vi "Open Playback Files Cropping.vi"(8 "error in (no error)":errorcluster, 11 "Frame Grabber Data In":T1={"Camera Session"="", "Frame"=refnum, "AVI Refnum"=refnum, "Codecs"=[], "Frame number"=0, "Tracking File Refnum"=refnum, "Tick Count"=0, "Probe Object"=refnum, "Playback Probe Data"=[], "Rigid Body"={"Position"={"x (mm)"=0.0, "y (mm)"=0.0, "z (mm)"=0.0}, "Orientation"={"Pitch (rad)"=0.0, "Yaw (rad)"=0.0, "Roll (rad)"=0.0}, "Quaternion"={"qx"=0.0, "qy"=0.0, "qz"=0.0, "qw"=0.0}, "Tracked?"=FALSE}, "Total no frames playback"=0, "Video FPS"=0.0, "Camera connected?"=FALSE, "Scene"=refnum, "Cropped Frame"=refnum, "Tracker FPS"=0.0, "Crop ROI"=[], "Presentation Values"=[], "Elapsed time (ms)"=0, "Camera frames playback"=0, "Refnums"={"Live Refnum"=refnum, "Record Refnum"=refnum, "Recording Settings Refnum"=refnum, "Playback Refnum"=refnum, "Frame Slider Refnum"=refnum, "Pause Refnum"=refnum, "Home Refnum"=refnum, "Crop Refnum"=refnum, "Clear Crop Refnum"=refnum, "stop refnum"=refnum, "Playback Rate Refnum"=refnum, "Operator Settings Refnums"=refnum, "Presentation Refnum"=refnum, "Gestation Refnum"=refnum, "Connection Settings Refnum"=refnum, "Crop Time Frame Slider Refnum"=refnum, "Cancel Save Refnum"=refnum}, "Dimensions"={"Probe Dimensions"={"Probe Width"=0.0, "Probe Depth"=1.0, "Probe Height"=0.0}, "Room Dimensions"={"Room Width"=0.0, "Room Depth"=0.0, "Room Height"=0.0}}, "Playback Data As Strings"=[], "Cropped Tracking File Refnum"=refnum, "Cropped AVI Refnum"=refnum, "Header"=[]}) -> (0 "error out":errorcluster, 1 "Playback Video":path, 2 "both exist and open?":bool, 3 "Frame Grabber Data Out":T1={"Camera Session"="", "Frame"=refnum, "AVI Refnum"=refnum, "Codecs"=[], "Frame number"=0, "Tracking File Refnum"=refnum, "Tick Count"=0, "Probe Object"=refnum, "Playback Probe Data"=[], "Rigid Body"={"Position"={"x (mm)"=0.0, "y (mm)"=0.0, "z (mm)"=0.0}, "Orientation"={"Pitch (rad)"=0.0, "Yaw (rad)"=0.0, "Roll (rad)"=0.0}, "Quaternion"={"qx"=0.0, "qy"=0.0, "qz"=0.0, "qw"=0.0}, "Tracked?"=FALSE}, "Total no frames playback"=0, "Video FPS"=0.0, "Camera connected?"=FALSE, "Scene"=refnum, "Cropped Frame"=refnum, "Tracker FPS"=0.0, "Crop ROI"=[], "Presentation Values"=[], "Elapsed time (ms)"=0, "Camera frames playback"=0, "Refnums"={"Live Refnum"=refnum, "Record Refnum"=refnum, "Recording Settings Refnum"=refnum, "Playback Refnum"=refnum, "Frame Slider Refnum"=refnum, "Pause Refnum"=refnum, "Home Refnum"=refnum, "Crop Refnum"=refnum, "Clear Crop Refnum"=refnum, "stop refnum"=refnum, "Playback Rate Refnum"=refnum, "Operator Settings Refnums"=refnum, "Presentation Refnum"=refnum, "Gestation Refnum"=refnum, "Connection Settings Refnum"=refnum, "Crop Time Frame Slider Refnum"=refnum, "Cancel Save Refnum"=refnum}, "Dimensions"={"Probe Dimensions"={"Probe Width"=0.0, "Probe Depth"=1.0, "Probe Height"=0.0}, "Room Dimensions"={"Room Width"=0.0, "Room Depth"=0.0, "Room Height"=0.0}}, "Playback Data As Strings"=[], "Cropped Tracking File Refnum"=refnum, "Cropped AVI Refnum"=refnum, "Header"=[]}, 5 "Number of Playback Frames":i32, 7 "Number of Camera Frames":u32)   [LabVIEW 2017]
uses:
  Controls/Frame Grabber Data.ctl
  <vilib>/userdefined/High Color/IMAQdx.ctl
  <vilib>/vision/Image Controls.llb/IMAQ Image.ctl
  <vilib>/vision/Avi.llb/IMAQ AVI2 Refnum.ctl
  Controls/Rigid Body Info.ctl
  Controls/Position.ctl
  Controls/Orientation.ctl
  Controls/Refnums.ctl
  Controls/Recording Settings.ctl
  Controls/Operator Settings.ctl
  Controls/Operator.ctl
  Controls/Dimensions.ctl
  Controls/Room Dimensions.ctl
  <vilib>/Utility/file.llb/Read Delimited Spreadsheet (string).vi
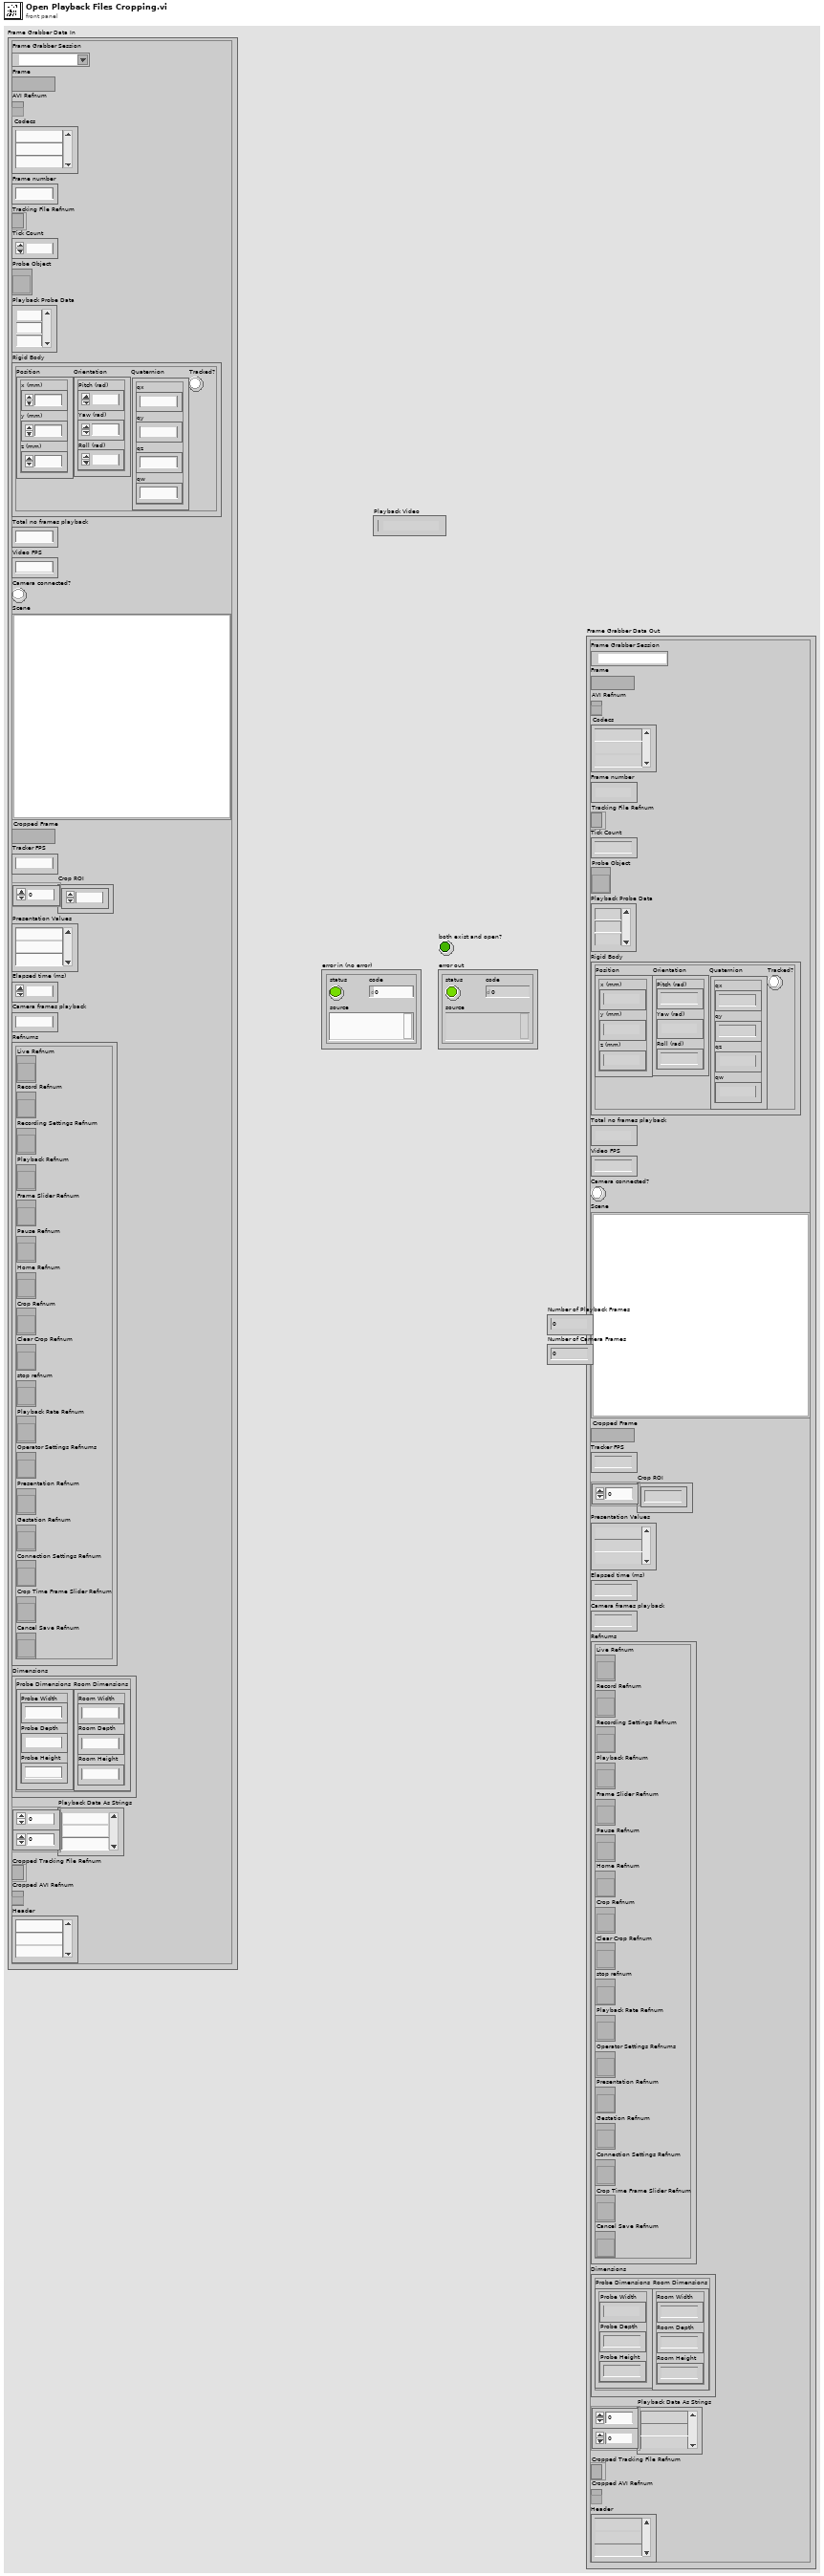
[diagram p1: front panel]
types:
  T1 = typedef "Frame Grabber Data.ctl" = cluster{"Camera Session":T2, "Frame":T3, "AVI Refnum":T4, "Codecs":string[], "Frame number":u32, "Tracking File Refnum":refnum<file>, "Tick Count":u32, "Probe Object":refnum<vi>, "Playback Probe Data":dbl[][], "Rigid Body":T5, "Total no frames playback":i32, "Video FPS":dbl, "Camera connected?":bool, "Scene":refnum<vi>, "Cropped Frame":T3, "Tracker FPS":dbl, "Crop ROI":i32[], "Presentation Values":string[], "Elapsed time (ms)":u32, "Camera frames playback":u32, "Refnums":T8, "Dimensions":T9, "Playback Data As Strings":string[][], "Cropped Tracking File Refnum":refnum<file>, "Cropped AVI Refnum":T4, "Header":string[]}
  T2 = typedef "IMAQdx.ctl" = refnum<k21>
  T3 = typedef "IMAQ Image.ctl" = refnum<image>
  T4 = typedef "IMAQ AVI2 Refnum.ctl" = refnum<k20>
  T5 = typedef "Rigid Body Info.ctl" = cluster{"Position":T6, "Orientation":T7, "Quaternion":cluster{"qx":sgl, "qy":sgl, "qz":sgl, "qw":sgl}, "Tracked?":bool}
  T6 = typedef "Position.ctl" = cluster{"x (mm)":sgl, "y (mm)":sgl, "z (mm)":sgl}
  T7 = typedef "Orientation.ctl" = cluster{"Pitch (rad)":sgl, "Yaw (rad)":sgl, "Roll (rad)":sgl}
  T8 = typedef "Refnums.ctl" = cluster{"Live Refnum":refnum<vi>, "Record Refnum":refnum<vi>, "Recording Settings Refnum":refnum<vi>, "Playback Refnum":refnum<vi>, "Frame Slider Refnum":refnum<vi>, "Pause Refnum":refnum<vi>, "Home Refnum":refnum<vi>, "Crop Refnum":refnum<vi>, "Clear Crop Refnum":refnum<vi>, "stop refnum":refnum<vi>, "Playback Rate Refnum":refnum<vi>, "Operator Settings Refnums":refnum<vi>, "Presentation Refnum":refnum<vi>, "Gestation Refnum":refnum<vi>, "Connection Settings Refnum":refnum<vi>, "Crop Time Frame Slider Refnum":refnum<vi>, "Cancel Save Refnum":refnum<vi>}
  T9 = typedef "Dimensions.ctl" = cluster{"Probe Dimensions":cluster{"Probe Width":sgl, "Probe Depth":sgl, "Probe Height":sgl}, "Room Dimensions":T10}
  T10 = typedef "Room Dimensions.ctl" = cluster{"Room Width":dbl, "Room Depth":dbl, "Room Height":dbl}
  T11 = enum16{"open", "replace", "create", "open or create", "replace or create", "replace or create with confirmation"}
  T12 = cluster{"Width":u32, "Height":u32, "Frames Per Second":u32, "Codec":string, "Has Data":bool}
  T13 = cluster{"Scale.Range:Minimum":i32, "Number of Frames":i32, "Scale.Range:Minimum":i32}
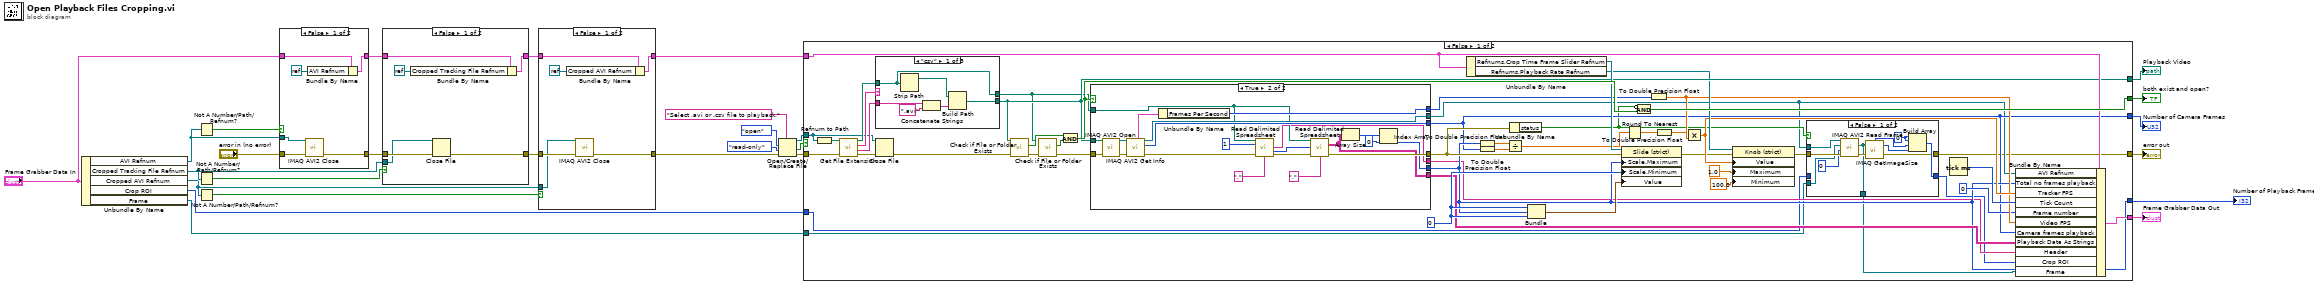
[diagram p0: block diagram]
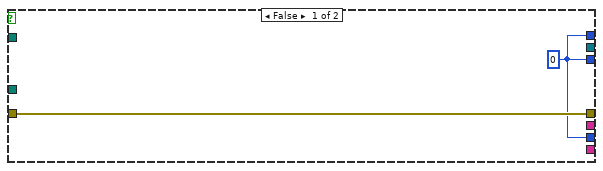
[diagram p6: hidden frame]
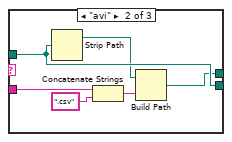
[diagram p7: hidden frame]
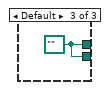
[diagram p8: hidden frame]
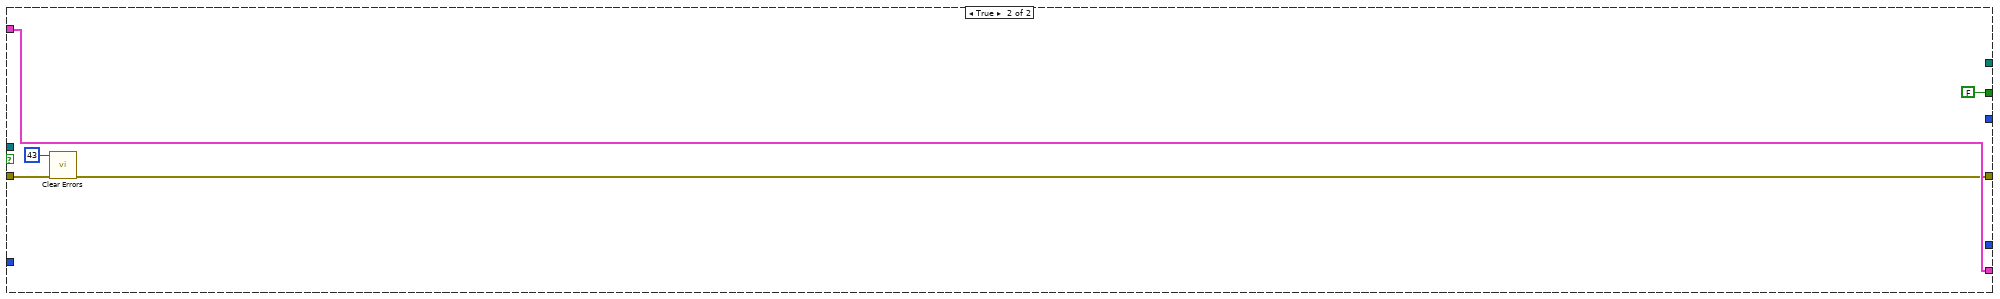
[diagram p9: hidden frame]
diagram:
  n1 = Unbundle By Name("Frame Grabber Data In") -> ("AVI Refnum"=w9:T4, "Cropped Tracking File Refnum"=w10:refnum<file>, "Cropped AVI Refnum"=w5:T4, "Crop ROI"=w2:i32[], "Frame"=w1:T3)
  n2 = Not A Number/Path/Refnum?(number/path/refnum=w9) -> (NaN/Path/Refnum?=w14:bool)
  n3 = Not A Number/Path/Refnum?(number/path/refnum=w10) -> (NaN/Path/Refnum?=w17:bool)
  n4 = Not A Number/Path/Refnum?(number/path/refnum=w5) -> (NaN/Path/Refnum?=w16:bool)
  n5 = case shown="False" w14 {
    tunnel: "error in (no error)" -> [w34 w36]
    tunnel: [w33 w36] -> w12
    tunnel: "Frame Grabber Data In" -> [w32 w35]
    tunnel: w9 -> [w31 _]
    tunnel: [w30 w35] -> w8
    frame False {
      n6 = call "IMAQ AVI2 Close"("error in (no error)"=w34, "AVI Refnum"=w31) -> ("error out"=w33:errorcluster)  [unwired: 9 in]
      n7 = Bundle By Name(cluster=w32, "AVI Refnum"=refnum<k0> refnum) -> (w30:T1)
    }
    frame True {
    }
  }
  n8 = case shown="False" w17 {
    tunnel: w12 -> [w42 w44]
    tunnel: [w41 w44] -> w18
    tunnel: w8 -> [w40 w43]
    tunnel: w10 -> [w39 _]
    tunnel: [w37 w43] -> w7
    frame False {
      n9 = Bundle By Name(cluster=w40, "Cropped Tracking File Refnum"=refnum<k0> refnum) -> (w37:T1)
      n10 = Close File(refnum=w39, error in=w42) -> (error out=w41:errorcluster)  [unwired: 1 out]
    }
    frame True {
    }
  }
  n11 = case shown="False" w16 {
    tunnel: w18 -> [w50 w52]
    tunnel: [w49 w52] -> w15
    tunnel: w7 -> [w48 w51]
    tunnel: [w47 w51] -> w6
    tunnel: w5 -> [w45 _]
    frame False {
      n12 = Bundle By Name(cluster=w48, "Cropped AVI Refnum"=refnum<k0> refnum) -> (w47:T1)
      n13 = call "IMAQ AVI2 Close"("error in (no error)"=w50, "AVI Refnum"=w45) -> ("error out"=w49:errorcluster)  [unwired: 9 in]
    }
    frame True {
    }
  }
  n14 = Open/Create/Replace File(error in=w15, prompt="Select .avi or .csv file to playback.", operation (0:open)=T11."open", access (0:read/write)=enum16{"read/write", "read-only", "write-only"}."read-only") -> (refnum out=w27:refnum<file>, cancelled=w21:bool, error out=w28:errorcluster)  [unwired: 2 in]
  n15 = case shown="False" w21 {
    tunnel: w28 -> [w100 w153]
    tunnel: w27 -> [w85 _]
    tunnel: w6 -> [w90 w155]
    tunnel: [w94 FALSE] -> w23
    tunnel: [w93 w155] -> w22
    tunnel: [w83 _] -> w20
    tunnel: [w57 w151] -> w19
    tunnel: [w66 _] -> w4
    tunnel: [w65 _] -> w3
    tunnel: w2 -> [w61 _]
    tunnel: w1 -> [w58 _]
    frame False {
      w69 = 0 ("Scale.Range:Minimum")
      n16 = Refnum to Path(1:w85) -> (0:w99:path)
      n17 = call <vilib>:"Get File Extension.vi"("error in (no error)"=w100, "file"=w99) -> ("error out"=w86:errorcluster, "filename without extension"=w97:string, "lowercase file extension"=w98:string, "dup file"=w96:path)  [unwired: 5 in, 1 out]
      n18 = case shown="\"csv\"" w98 {
        tunnel: w97 -> [w143 w148 _]
        tunnel: w96 -> [w140 w147 _]
        tunnel: [w138 w147 w150] -> w83
        tunnel: [w140 w144 w150] -> w80
        frame "csv" {
          n19 = Strip Path(path=w140) -> (stripped path=w141:path)  [unwired: 1 out]
          n20 = Concatenate Strings(w143, ".avi" ("string")) -> (w139:string)
          n21 = Build Path(base path=w141, name or relative path=w139) -> (appended path=w138:path)
        }
        frame "avi" {
          n22 = Strip Path(path=w147) -> (stripped path=w146:path)  [unwired: 1 out]
          n23 = Concatenate Strings(w148, ".csv" ("string")) -> (w145:string)
          n24 = Build Path(base path=w146, name or relative path=w145) -> (appended path=w144:path)
        }
        frame Default {
          w150 = path "" ("dup file")
        }
      }
      n25 = Close File(refnum=w85, error in=w86) -> (error out=w84:errorcluster)  [unwired: 1 out]
      n26 = call <vilib>:"Check if File or Folder Exists.vi"("error in (no error)"=w84, "path"=w83) -> ("error out"=w78:errorcluster, "file or folder exists?"=w82:bool)  [unwired: 7 in, 1 out]
      n27 = call <vilib>:"Check if File or Folder Exists.vi"("error in (no error)"=w78, "path"=w80) -> ("error out"=w81:errorcluster, "file or folder exists?"=w79:bool)  [unwired: 7 in, 1 out]
      n28 = And(x=w82, y=w79) -> (x .and. y?=w95:bool)
      n29 = case shown="True" w95 {
        tunnel: w81 -> [w116 w131]
        tunnel: w83 -> [_ w137]
        tunnel: [w116 w124] -> w91
        tunnel: [_ w134] -> w59
        tunnel: w80 -> [_ w127]
        tunnel: [w115 w128] -> w65
        tunnel: [w115 w132] -> w87
        tunnel: [w115 w122] -> w66
        tunnel: [_ w123] -> w68
        tunnel: [_ w118] -> w64
        frame False {
          w115 = 0 ("Number of Frames")
        }
        frame True {
          n30 = call "IMAQ AVI2 Open"("error in (no error)"=w131, "AVI File Path"=w137) -> ("error out"=w136:errorcluster, "AVI Refnum"=w135:T4)  [unwired: 8 in]
          n31 = call "IMAQ AVI2 Get Info"("error in (no error)"=w136, "AVI Refnum"=w135) -> ("error out"=w130:errorcluster, "Number of Frames"=w128:u32, "AVI Refnum (duplicate)"=w134:T4, "Frame Data"=w133:T12)  [unwired: 5 in, 1 out]
          n32 = Unbundle By Name(w133) -> ("Frames Per Second"=w132:u32)
          n33 = call-poly <vilib>:"Read Delimited Spreadsheet.vi"("file path (dialog if empty)"=w127, "number of rows (all:-1)"=1, "error in (no error)"=w130, "delimiter (\\t)"="," ("delimiter (\\t)")) -> ("first row"=w118:string[], "mark after read (chars.)"=w125:i32, "error out"=w126:errorcluster)  [unwired: 6 in, 3 out]
          n34 = call-poly <vilib>:"Read Delimited Spreadsheet.vi"("file path (dialog if empty)"=w127, "start of read offset (chars.:0)"=w125, "error in (no error)"=w126, "delimiter (\\t)"="," ("delimiter (\\t)")) -> ("all rows"=w123:string[][], "error out"=w124:errorcluster)  [unwired: 6 in, 4 out]
          n35 = Array Size(array=w123) -> (size(s)=w121:i32[])
          n36 = Index Array(array=w121, index=0) -> (element=w122:i32)
        }
      }
      n37 = Unbundle By Name(w90) -> ("Refnums.Crop Time Frame Slider Refnum"=w89:refnum<vi>, "Refnums.Playback Rate Refnum"=w77:refnum<vi>)
      n38 = To Double Precision Float(number=w66) -> (double precision float=w54:dbl)
      n39 = To Double Precision Float(number=w65) -> (double precision float=w53:dbl)
      n40 = Divide(x=w54, y=w53) -> (x/y=w88:dbl)
      n41 = Unbundle By Name(w91) -> ("status"=w63:bool)
      n42 = Bundle("Scale.Range:Minimum"=w69, "Number of Frames"=w66, "Scale.Range:Minimum"=w69) -> (w70:T13)  [unwired: 1 in]
      n43 = property class="Slide (strict)"(reference=w89, error in=w91, "Scale.Maximum"=w66, "Scale.Minimum"=w69, "Value"=w70) -> (error out=w75:errorcluster)  [unwired: 1 out]
      n44 = Round To Nearest(number=w88) -> (nearest integer value=w55:dbl)
      n45 = Compound Arithmetic op=AND(invert w63, w95) -> (w94:bool)
      n46 = To Double Precision Float(number=w87) -> (double precision float=w72:dbl)
      n47 = To Double Precision Float(number=w55) -> (double precision float=w71:dbl)
      n48 = Multiply(x=w71, y=w72) -> (x*y=w76:dbl)
      n49 = property class="Knob (strict)"(reference=w77, error in=w75, "Value"=w76, "Maximum"=1.0 ("Data Entry Limits:Maximum"), "Minimum"=100.0 ("Data Entry Limits:Minimum")) -> (error out=w62:errorcluster)  [unwired: 1 out]
      n50 = case shown="False" w63 {
        tunnel: w62 -> [w111 w113]
        tunnel: w61 -> [_ w114]
        tunnel: [w106 w114] -> w60
        tunnel: w59 -> [w105 _]
        tunnel: w58 -> [w103 w112]
        tunnel: [w102 w113] -> w57
        tunnel: [w101 w112] -> w56
        frame False {
          w107 = 0 ("element")
          n51 = call "IMAQ AVI2 Read Frame"("error in (no error)"=w111, "Frame Number"=u32 0, "Image"=w103, "AVI Refnum"=w105) -> ("error out"=w110:errorcluster, "Image Out"=w101:T3)  [unwired: 5 in, 1 out]
          n52 = call "IMAQ GetImageSize"("Image"=w101, "error in (no error)"=w110) -> ("Y Resolution"=w109:i32, "X Resolution"=w108:i32, "error out"=w102:errorcluster)  [unwired: 2 in]
          n53 = Build Array(w107, w107, w108, w109) -> (w106:i32[])
        }
        frame True {
        }
      }
      n54 = Tick Count (ms)() -> (millisecond timer value=w92:u32)
      n55 = Bundle By Name(cluster=w90, "AVI Refnum"=w59, "Total no frames playback"=w66, "Tracker FPS"=w76, "Tick Count"=w92, "Frame number"=u32 0, "Video FPS"=w72, "Camera frames playback"=w65, "Playback Data As Strings"=w68, "Header"=w64, "Crop ROI"=w60, "Frame"=w56) -> (w93:T1)
    }
    frame True {
      n56 = call <vilib>:"Clear Errors.vi"("error in (no error)"=w153, "specific error code to clear (0: all)"=43) -> ("error out"=w151:errorcluster)  [unwired: 4 in, 1 out]
    }
  }
  "both exist and open?" <- w23
  "Frame Grabber Data Out" <- w22
  "Playback Video" <- w20
  "error out" <- w19
  "Number of Playback Frames" <- w4
  "Number of Camera Frames" <- w3
